vi "getChildren.vi"(0 "reference":refnum<class "AbstractNode.lvclass">, 5 "error in (no error)":errorcluster) -> (14 "reference out":refnum<class "AbstractNode.lvclass">, 15 "children":refnum<class "AbstractNode.lvclass">[](array[class]), 17 "Refs":u32[](array[numeric]), 19 "error out":errorcluster)   [LabVIEW 2012, in "AbstractNode.lvclass"]
doc: "public List getChildren()"
uses:
  <resource>/Framework/Providers/Open_GDS/UML/AbstractNode_class/AbstractNode.lvclass
  <resource>/Framework/Providers/Open_GDS/UML/AbstractNode_class/AbstractNode.lvclass/AbstractNode.ctl
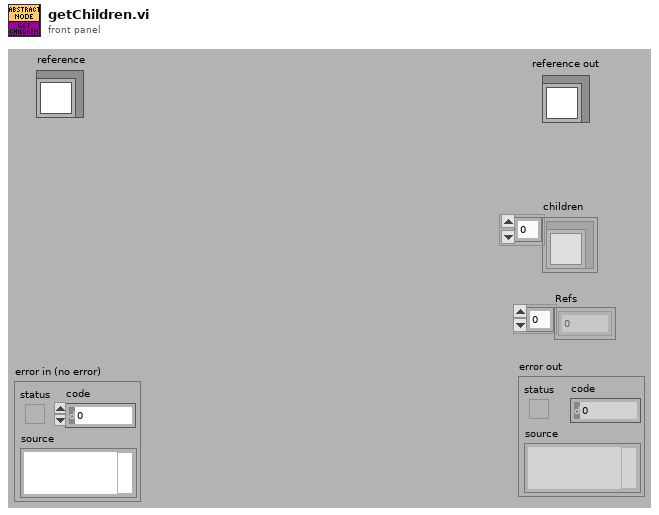
[diagram p1: front panel]
types:
  T1 = typedef "AbstractNode.lvclass/ObjectAttributes.ctl" = cluster{"parent":refnum<class "AbstractNode.lvclass">, "children":refnum<class "AbstractNode.lvclass">[], "Hidden":bool}
  T2 = typedef "AbstractNode.lvclass/ObjectReference.ctl" = refnum<k1>
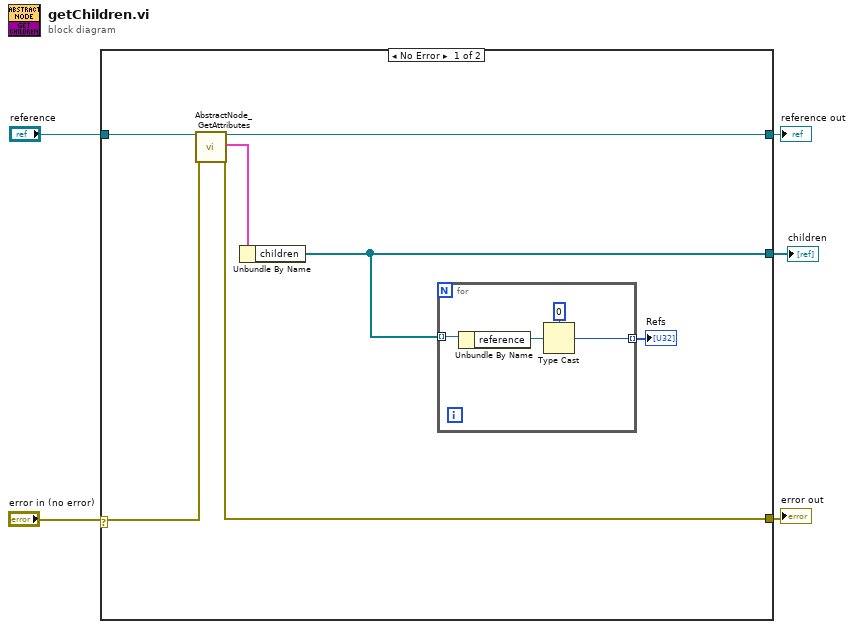
[diagram p0: block diagram]
diagram:
  n1 = case shown="No Error" "error in (no error)" {
    selector: "error in (no error)" -> [w9 w17]
    tunnel: "reference" -> [w12 w18]
    tunnel: [w11 w17] -> w4
    tunnel: [w10 w18] -> w3
    tunnel: [w7 _] -> w1
    frame No Error {
      n2 = call <resource>:"AbstractNode_GetAttributes.vi"("reference in"=w12, "error in (no error)"=w9) -> ("reference out"=w10:refnum<class "AbstractNode.lvclass">, "Attributes"=w8:T1, "error out"=w11:errorcluster)  [unwired: 15 out]
      n3 = Unbundle By Name(w8) -> ("children"=w7:refnum<class "AbstractNode.lvclass">[])
      n4 = for {
        tunnel: w7 -> [w15] mode=indexing
        tunnel: [w13] -> w6 mode=indexing
        n5 = Unbundle By Name(w15) -> ("reference"=w14:T2)
        n6 = Type Cast(type=u32 0, x=w14) -> (*(type *) &x=w13:u32)
      }
      "Refs" <- w6
    }
    frame Error {
    }
  }
  "reference out" <- w3
  "error out" <- w4
  "children" <- w1
